vi "set_corners.vi"(8 "error in (no error)":errorcluster, 9 "corner 2":refnum<class "SpaceVector.lvclass">, 10 "corner 1":refnum<class "SpaceVector.lvclass">, 11 "RoiGeneric in":refnum<class "RoiGeneric.lvclass">) -> (0 "error out":errorcluster, 3 "RoiGeneric out":refnum<class "RoiGeneric.lvclass">)   [LabVIEW 2010]
uses:
  common/classes/Box/Box/Box.lvclass
  RoiGeneric.lvclass
  common/classes/SpaceVector/SpaceVector/SpaceVector.lvclass
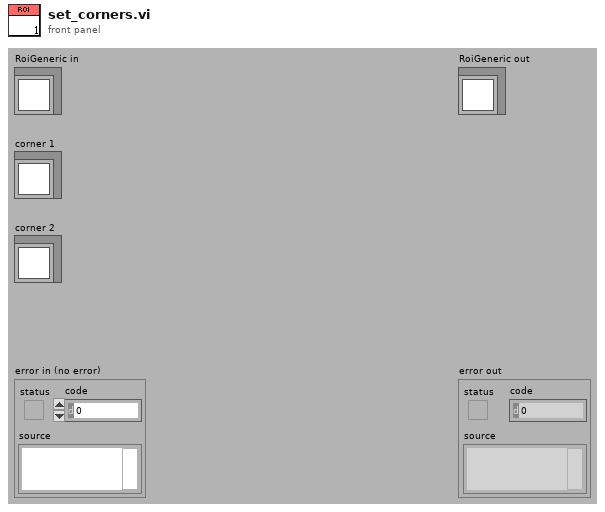
[diagram p1: front panel]
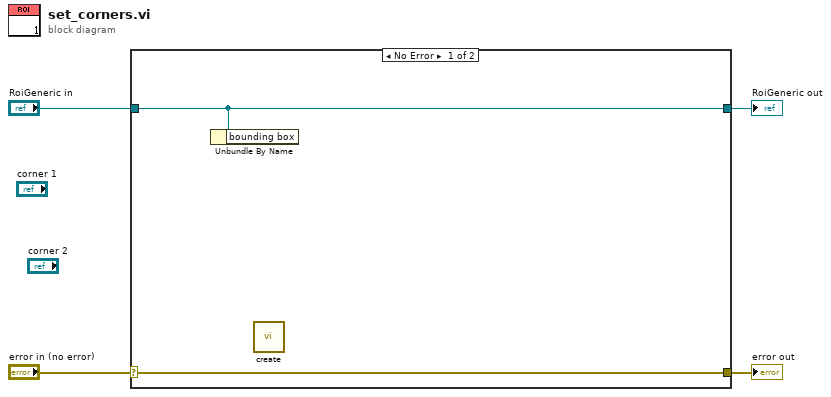
[diagram p0: block diagram]
diagram:
  n1 = case shown="No Error" "error in (no error)" {
    selector: "error in (no error)" -> [w6 w8]
    tunnel: [w6 w8] -> w3
    tunnel: [w5 w7] -> w1
    tunnel: "RoiGeneric in" -> [w5 w7]
    frame No Error {
      n2 = Unbundle By Name(w5) -> ()  [unwired: 1 out]
      n3 = call "create.vi"() -> ()  [unwired: 10 in, 2 out]
    }
    frame Error {
    }
  }
  "error out" <- w3
  "RoiGeneric out" <- w1
